vi "Basic XY 1D Data Buffer.vi"(0 "Inputs":dbl[](array[numeric]), 7 "Buffer Size":i32=5000, 11 "Reset":bool, 13 "Timestamps":dbl[](array[numeric])) -> (4 "Data":cluster{"Data":cluster{"Time":dbl, "Y":dbl}[]}[](array[cluster]))   [LabVIEW 2011]
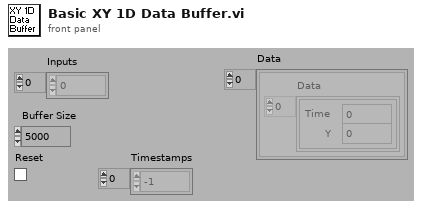
[diagram p1: front panel]
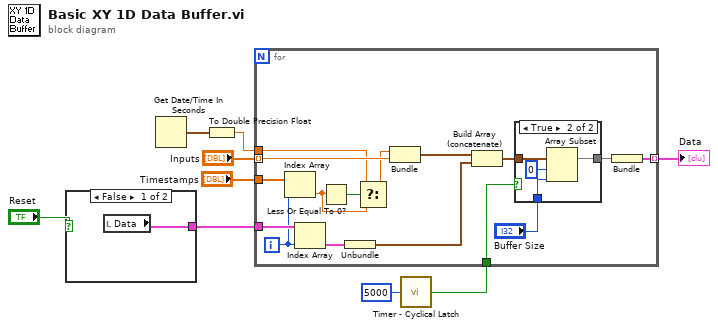
[diagram p0: block diagram]
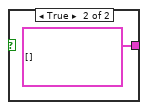
[diagram p2: hidden frame]
diagram:
  n1 = case shown="False" "Reset" {
    tunnel: [w10 cluster{cluster{dbl, dbl}[]}[] [] ("XY Graph 2")] -> w9
    frame False {
      n2 = local read "Data"() -> (w10:cluster{"Data":cluster{"Time":dbl, "Y":dbl}[]}[])
    }
    frame True {
    }
  }
  n3 = Get Date/Time In Seconds() -> (seconds since 1Jan1904=w6:timestamp)
  n4 = To Double Precision Float(number=w6) -> (double precision float=w5:dbl)
  n5 = call "Timer - Cyclical Latch.vi"("Timer (msec)"=u32 5000) -> ("Timer Trigger"=w2:bool)  [unwired: 14 in]
  n6 = for {
    tunnel: w9 -> [w27]
    tunnel: "Inputs" -> [w15] mode=indexing
    tunnel: [w25] -> w4 mode=indexing
    tunnel: w5 -> [w12]
    tunnel: w2 -> [w23]
    tunnel: "Timestamps" -> [w18]
    i -> [w17]
    n7 = Index Array(array=w18, index=w17) -> (element=w13:dbl)
    n8 = Index Array(array=w27, index=w17) -> (element=w26:cluster{"Data":cluster{"Time":dbl, "Y":dbl}[]})
    n9 = Less Or Equal To 0?(x=w13) -> (x <= 0?=w16:bool)
    n10 = Unbundle(w26) -> ("Data"=w20:cluster{"Time":dbl, "Y":dbl}[])
    n11 = Select(t=w12, s=w16, f=w13) -> (s? t:f=w14:dbl)
    n12 = Bundle("Numeric"=w14, "Numeric"=w15) -> (w21:cluster{"Numeric":dbl, "Numeric":dbl})  [unwired: 1 in]
    n13 = Build Array (concatenate)(w21, w20) -> (w24:cluster{"Time":dbl, "Y":dbl}[])
    n14 = case shown="True" w23 {
      tunnel: w24 -> [w28 w32]
      tunnel: [w28 w31] -> w22
      tunnel: "Buffer Size" -> [_ w29]
      frame False {
      }
      frame True {
        n15 = Array Subset(array=w32, index=0, length=w29) -> (w31:cluster{"Time":dbl, "Y":dbl}[])
      }
    }
    n16 = Bundle(w22) -> (w25:cluster{cluster{"Time":dbl, "Y":dbl}[]})  [unwired: 1 in]
  }
  "Data" <- w4
